vi "Puff_using_ADAM_Ch.vi"() -> (5 "Plug in titles":string[](array[string]), 7 "Plug in values":string[](array[string]))   [LabVIEW 2011]
uses:
  Controls/Post_Process.ctl
  Globals/Meas_global.vi
  Globals/Dynamic_call_global.ph.vi
panel:
  in  "Source Off Wait":u32=7000
  out "Block Number currently taking":i32=16
  out "No Of Blocks":i32=16
  in  "Source on Wait":u32=7000
  out "Case Currently On":string="Set Acquisition interlock"
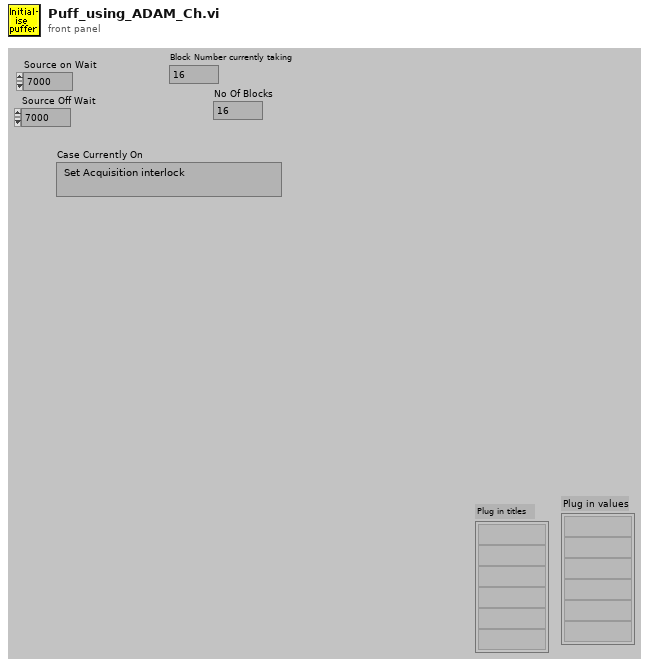
[diagram p1: front panel]
types:
  T1 = typedef "Post_Process.ctl" = enum16{"Take New Data", "Post Process Raw Data File"}
  T2 = typedef "Rendezvous RefNum" = refnum<k1>
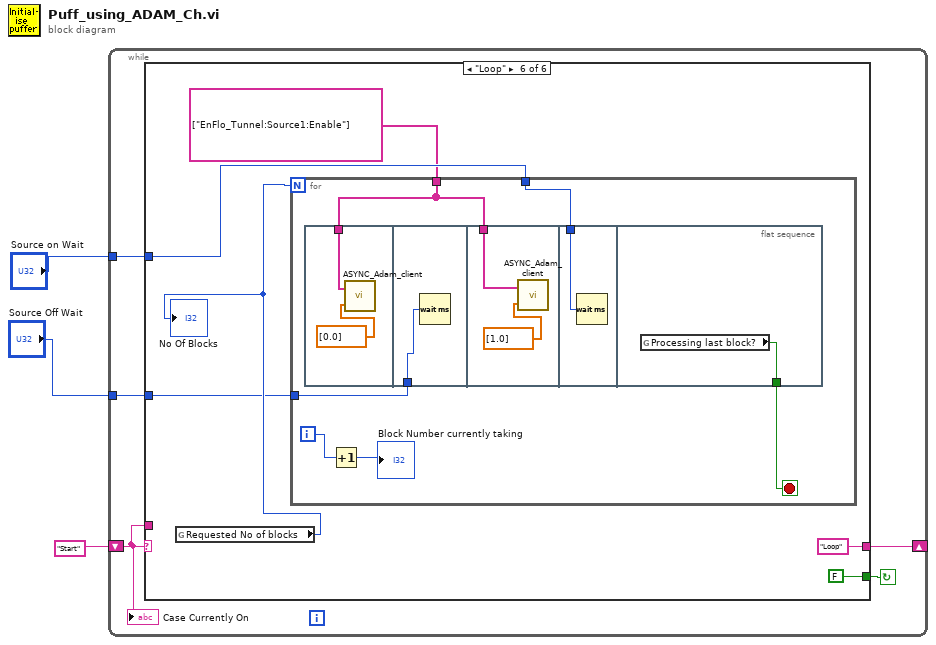
[diagram p0: block diagram]
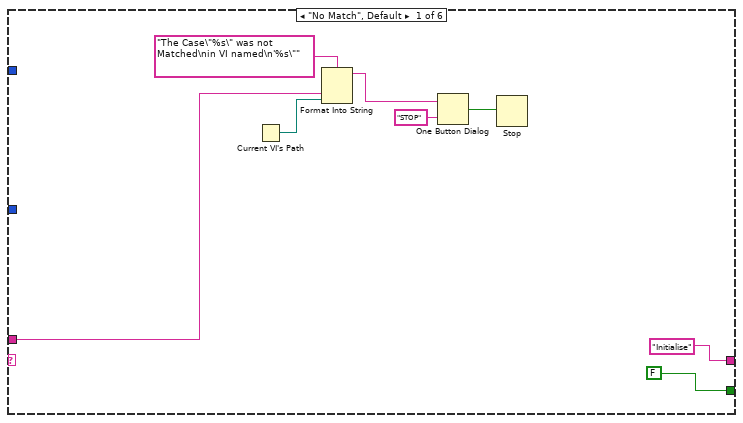
[diagram p2: hidden frame]
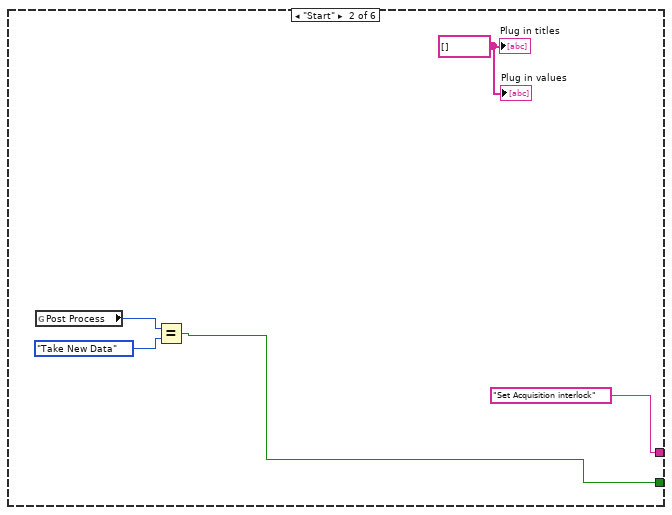
[diagram p3: hidden frame]
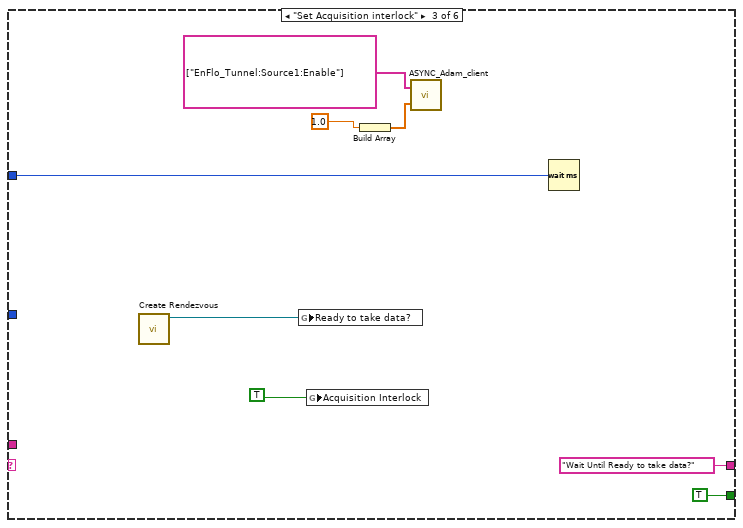
[diagram p4: hidden frame]
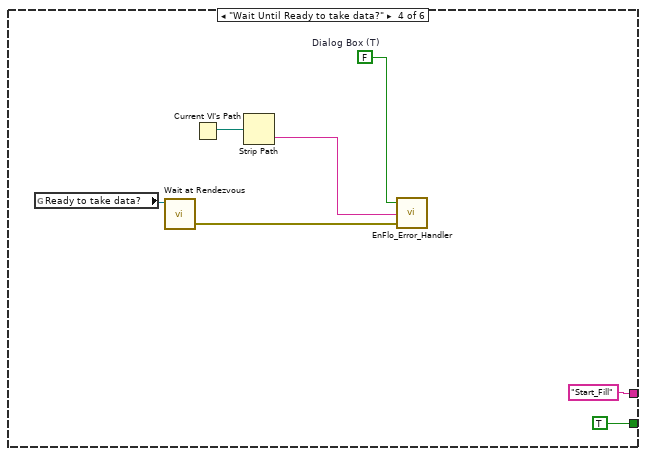
[diagram p5: hidden frame]
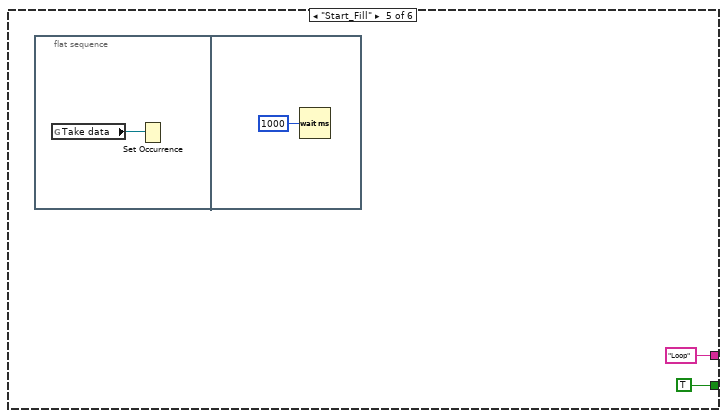
[diagram p6: hidden frame]
diagram:
  n1 = while {
    shift-left: "Start" -> [w6]
    shift-right: [w7] -> _
    tunnel: "Source on Wait" -> [w5]
    tunnel: "Source Off Wait" -> [w4]
    stop <- w8 continue-if-true
    n2 = case shown="\"Loop\"" w6 {
      tunnel: [FALSE w17 TRUE ("Command Found") TRUE ("Command Found") TRUE ("Command Found") FALSE ("Command Found")] -> w8
      tunnel: ["Initialise" "Set Acquisition interlock" "Wait Until Ready to take data?" "Start_Fill" "Loop" "Loop"] -> w7
      tunnel: w6 -> [w11 _ _ _ _ _]
      tunnel: w5 -> [_ _ w22 _ _ w44]
      tunnel: w4 -> [_ _ _ _ _ w41]
      frame "No Match", Default {
        n3 = Current VI's Path() -> (path=w10:path)
        n4 = Format Into String(format string="The Case\"%s\" was not Matched\nin VI named\n'%s\"" ("Format String"), w11, w10) -> (resulting string=w14:string)  [unwired: 2 in, 1 out]
        n5 = One Button Dialog(message=w14, button name ("OK")="STOP") -> (true=w12:bool)
        n6 = Stop(stop? (T)=w12) -> ()
      }
      frame "Start" {
        w18 = string[] [] ("Plug in titles")
        n7 = global read "Meas_global.vi" "Post Process"() -> (w19:T1)
        n8 = Equal?(x=w19, y=Post_Process."Take New Data" ("Post Process")) -> (x = y?=w17:bool)
        "Plug in values" <- w18
        "Plug in titles" <- w18
      }
      frame "Set Acquisition interlock" {
        n9 = call <vilib>:"Create Rendezvous.vi"() -> ("rendezvous"=w26:T2)  [unwired: 5 in, 2 out]
        n10 = global write "Dynamic_call_global.ph.vi" "Ready to take data?"(w26) -> ()
        n11 = global write "Dynamic_call_global.ph.vi" "Acquisition Interlock"(TRUE ("Remote control")) -> ()
        n12 = Build Array(1.0 ("New Value")) -> (w25:dbl[])
        n13 = call "ASYNC_Adam_client.vi"("Values"=w25, "Channel Names"=string[] ["EnFlo_Tunnel:Source1:Enable"] ("appended array")) -> ()  [unwired: 2 out]
        n14 = Wait (ms)(milliseconds to wait=w22) -> ()  [unwired: 1 out]
      }
      frame "Wait Until Ready to take data?" {
        w32 = FALSE  # Dialog Box (T)
        n15 = global read "Dynamic_call_global.ph.vi" "Ready to take data?"() -> (w35:T2)
        n16 = call <vilib>:"Wait at Rendezvous.vi"("rendezvous"=w35) -> ("error out"=w33:errorcluster)  [unwired: 4 in, 2 out]
        n17 = Current VI's Path() -> (path=w31:path)
        n18 = Strip Path(path=w31) -> (name=w30:string)  [unwired: 1 out]
        n19 = call "EnFlo_Error_Handler.vi"("error in (no error)"=w33, "Error Type"=w30, "Dialog Box (T)"=w32) -> ()  [unwired: 3 out]
      }
      frame "Start_Fill" {
        n20 = flat-sequence {
          frame #0 {
            n21 = global read "Dynamic_call_global.ph.vi" "Take data"() -> (w39:refnum<k4>)
            n22 = Set Occurrence(w39) -> ()
          }
          frame #1 {
            n23 = Wait (ms)(milliseconds to wait=u32 1000) -> ()  [unwired: 1 out]
          }
        }
      }
      frame "Loop" {
        n24 = global read "Meas_global.vi" "Requested No of blocks"() -> (w42:i32)
        "No Of Blocks" <- w42
        n25 = for {
          N: w42 -> [_]
          tunnel: w44 -> [w51]
          tunnel: string[] ["EnFlo_Tunnel:Source1:Enable"] ("appended array") -> [w52]
          tunnel: w41 -> [w48]
          i -> [w50]
          stop <- w47 stop-if-true
          n26 = flat-sequence {
            tunnel: w52 -> [w54]
            tunnel: w48 -> [w55]
            tunnel: w52 -> [w57]
            tunnel: w51 -> [w58]
            tunnel: [w59] -> w47
            frame #0 {
              n27 = call "ASYNC_Adam_client.vi"("Values"=dbl[] [0.0] ("appended array"), "Channel Names"=w54) -> ()  [unwired: 2 out]
            }
            frame #1 {
              n28 = Wait (ms)(milliseconds to wait=w55) -> ()  [unwired: 1 out]
            }
            frame #2 {
              n29 = call "ASYNC_Adam_client.vi"("Values"=dbl[] [1.0] ("appended array"), "Channel Names"=w57) -> ()  [unwired: 2 out]
            }
            frame #3 {
              n30 = Wait (ms)(milliseconds to wait=w58) -> ()  [unwired: 1 out]
            }
            frame #4 {
              n31 = global read "Meas_global.vi" "Processing last block?"() -> (w59:bool)
            }
          }
          n32 = Increment(x=w50) -> (x+1=→"Block Number currently taking":i32)
        }
      }
    }
    "Case Currently On" <- w6
  }
